vi "Iterate-acquisition.vi"(8 "error in":errorcluster, 9 "Reset?":bool, 11 "Data ref. in":refnum<data-value>) -> (0 "error IO":errorcluster, 3 "Data ref.":refnum<data-value>)   [LabVIEW 2013, in "CameraVision.lvlib" / "CV-Main.lvclass"]
doc: "This function increases the layer/iteration number by one (+1)."
uses:
  CV-Main.lvclass
  CV-Main.lvclass/CV-Main.ctl
  Storage/CV-Storage.lvclass/CV-Storage.ctl
  Read Storage params.vi
  Storage/CV-Storage.lvclass
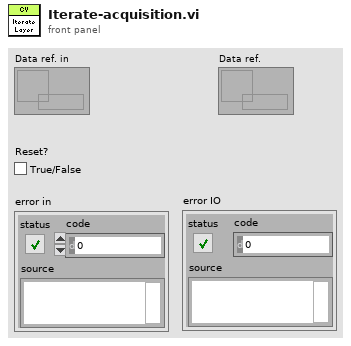
[diagram p1: front panel]
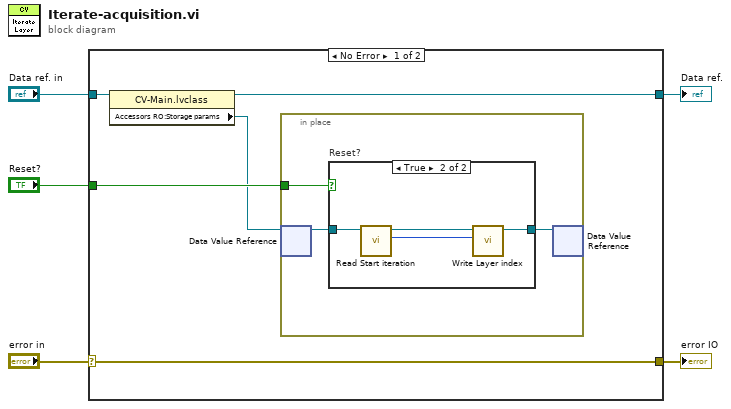
[diagram p0: block diagram]
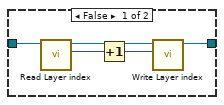
[diagram p2: hidden frame]
diagram:
  n1 = case shown="No Error" "error in" {
    selector: "error in" -> [w7 w24]
    tunnel: [w7 w24] -> w4
    tunnel: "Data ref. in" -> [w10 w23]
    tunnel: [w9 w23] -> w2
    tunnel: "Reset?" -> [w8 _]
    frame No Error {
      n2 = property class="CV-Main.lvclass"(reference=w10) -> (reference out=w9:refnum<data-value>, "Accessors RO:Storage params"=w6:refnum<data-value>)  [unwired: 1 in, 1 out]
      n3 = in-place {
        in-place-border: w8 -> [w13]
        n4 = in-place-dvr #1(w6) -> (w12:refnum<class "CV-Storage.lvclass">)  [unwired: 1 out]
        n5 = case "Reset?" shown="True" w13 {
          tunnel: [w14 w21] -> w11
          tunnel: w12 -> [w18 w22]
          frame False {
            n6 = call "Read Layer index.vi"("Storage params in"=w18) -> ("Iteration/layer index"=w17:u16, "Storage params out"=w16:refnum<class "CV-Storage.lvclass">)  [unwired: 8 in, 1 out]
            n7 = Increment(x=w17) -> (x+1=w15:u16)
            n8 = call "Write Layer index.vi"("Iteration/layer index"=w15, "Storage params in"=w16) -> ("Storage params out"=w14:refnum<class "CV-Storage.lvclass">)  [unwired: 8 in, 1 out]
          }
          frame True {
            n9 = call "Read Start iteration.vi"("Storage in"=w22) -> ("Start iteration/layer"=w19:u16, "Storage out"=w20:refnum<class "CV-Storage.lvclass">)  [unwired: 8 in, 1 out]
            n10 = call "Write Layer index.vi"("Iteration/layer index"=w19, "Storage params in"=w20) -> ("Storage params out"=w21:refnum<class "CV-Storage.lvclass">)  [unwired: 8 in, 1 out]
          }
        }
        n11 = in-place-dvr #1(w11) -> ()  [unwired: 2 out]
      }
    }
    frame Error {
    }
  }
  "error IO" <- w4
  "Data ref." <- w2
